vi "AI5_CurrentSense.vi"(8 "error in (no error)":errorcluster, 11 "Device":string="Dev1") -> (0 "error out":errorcluster, 3 "Current (Amps)":dbl=105.61954196628504 format="%0.2f")   [LabVIEW 2015]
uses:
  <vilib>/DAQmx/read.llb/DAQmx Read (Analog DBL 1Chan 1Samp).vi
  <vilib>/DAQmx/create/channels.llb/DAQmx Create Channel (AI-Voltage-Basic).vi
  <vilib>/DAQmx/miscellaneous.llb/DAQmx Fill In Error Info.vi
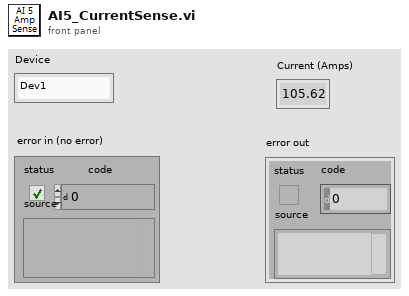
[diagram p1: front panel]
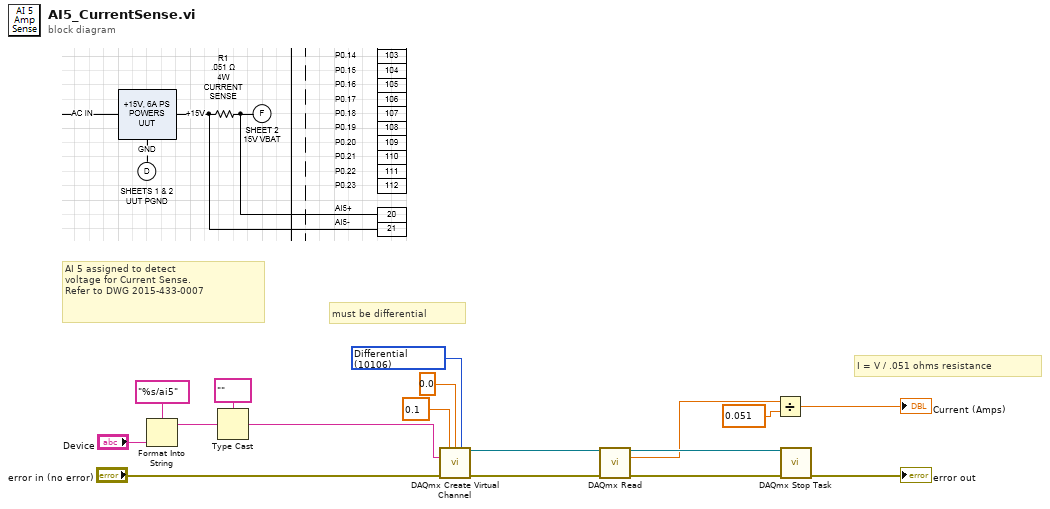
[diagram p0: block diagram]
diagram:
  w8 = 10106 items=["Default"=-1, "RSE"=10083, "NRSE"=10078, "Differential"=10106, "Pseudodifferential"=12529] ("input terminal configuration")
  # "must be differential"
  # "I = V / .051 ohms resistance"
  # "AI 5 assigned to detect\nvoltage for Current Sense.\nRefer to DWG 2015-433-0007"
  n1 = Format Into String(format string="%s/ai5", "Device") -> (resulting string=w5:string)  [unwired: 2 in, 1 out]
  n2 = Type Cast(type=tag "" ("lines"), x=w5) -> (*(type *) &x=w3:tag)
  n3 = call-poly <vilib>:"DAQmx Create Virtual Channel.vi"("maximum value"=0.1, "minimum value"=0.0, "input terminal configuration"=w8, "physical channels"=w3, "error in"="error in (no error)") -> ("task out"=w17:refnum<k21>, "error out"=w16:errorcluster)  [unwired: 9 in]
  n4 = call-poly <vilib>:"DAQmx Read.vi"("task/channels in"=w17, "error in"=w16) -> ("task out"=w14:refnum<k21>, "data"=w12:dbl, "error out"=w15:errorcluster)  [unwired: 11 in]
  n5 = Divide(x=w12, y=0.051 ("x")) -> (x/y=→"Current (Amps)":dbl)
  n6 = call <vilib>:"DAQmx Stop Task.vi"("task/channels in"=w14, "error in"=w15) -> ("error out"=→"error out":errorcluster)  [unwired: 12 in, 1 out]
